vi "LifetimeImageglobal.vi"(1 "Palette Number (gray)":T2(ring), 4 "min tau value":dbl format="%.2f", 5 "max tau value":dbl format="%.2f", 6 "input Image array":u8[][](array[numeric]), 7 "error in":errorcluster, 8 "Enum":T1(ring)) -> (0 "title":string, 2 "error out":errorcluster, 3 "New Image":T3)   [LabVIEW 2009]
uses:
  <vilib>/vision/Image Controls.llb/IMAQ Image.ctl
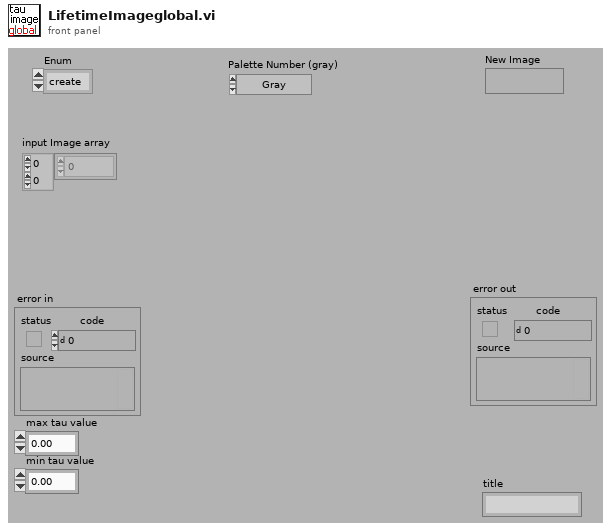
[diagram p1: front panel]
types:
  T1 = enum16{"create", "Input", "draw", "colorpal", "dump", "get", "kill"}
  T2 = enum32{"Gray", "Binary", "Gradient", "Rainbow", "Temperature"}
  T3 = typedef "IMAQ Image.ctl" = refnum<image>
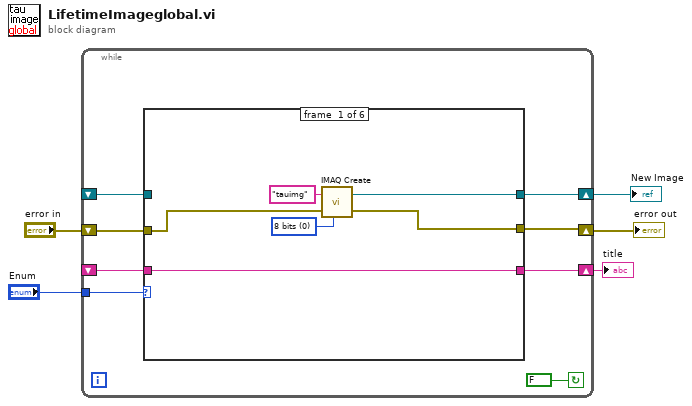
[diagram p0: block diagram]
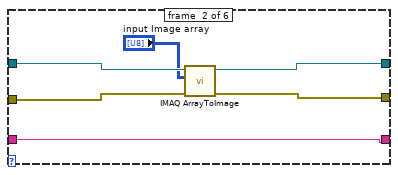
[diagram p2: hidden frame]
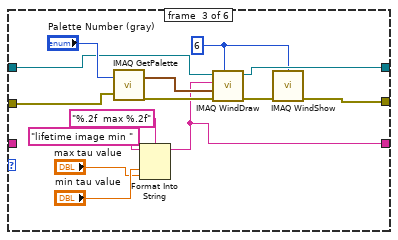
[diagram p3: hidden frame]
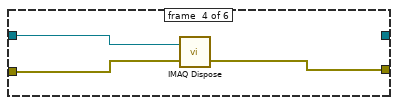
[diagram p4: hidden frame]
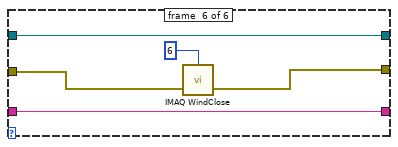
[diagram p6: hidden frame]
diagram:
  n1 = while {
    shift-right: [w11] -> w5
    shift-left: _ -> [w13]
    shift-right: [w10] -> w4
    shift-left: "error in" -> [w12]
    shift-right: [w9] -> w2
    shift-left: _ -> [w8]
    tunnel: "Enum" -> [w6]
    stop <- FALSE continue-if-true
    n2 = case shown="\"kill\"" w6 {
      tunnel: w13 -> [_ w23 w35 w42 w44 w49]
      tunnel: w12 -> [w16 w25 w39 w41 _ w47]
      tunnel: [w17 w22 w34 _ w44 w49] -> w11
      tunnel: [w15 w24 w32 w40 _ w46] -> w10
      tunnel: [w14 w20 w28 _ w43 w48] -> w9
      tunnel: w8 -> [w14 w20 _ _ w43 w48]
      frame #0 {
        w18 = u32 0 items=["8 bits", "16 bits", "Float", "Complex", "RGB", "HSL"] ("Image Type")
        n3 = call "IMAQ Create"("Image Name"="tauimg", "Image Type"=w18, "error in (no error)"=w16) -> ("New Image"=w17:T3, "error out"=w15:errorcluster)  [unwired: 2 in]
      }
      frame #1 {
        n4 = call "IMAQ ArrayToImage"("error in (no error)"=w25, "Image Pixels (U8)"="input Image array", "Image"=w23) -> ("error out"=w24:errorcluster, "Image Out"=w22:T3)  [unwired: 7 in]
      }
      frame #2 {
        w31 = 6 ("Window Number (0...15)")
        n5 = call "IMAQ GetPalette"("Palette Number (gray)"="Palette Number (gray)", "error in (no error)"=w39) -> ("Color Palette"=w36:cluster{"Red":u8, "Green":u8, "Blue":u8}[], "error out"=w37:errorcluster)  [unwired: 3 in]
        n6 = Format Into String(format string="%.2f  max %.2f", initial string="lifetime image min ", "min tau value", "max tau value") -> (resulting string=w28:string)  [unwired: 1 in, 1 out]
        n7 = call "IMAQ WindDraw"("Window Number (0...15)"=w31, "error in (no error)"=w37, "Color Palette"=w36, "Title"=w28, "Image"=w35) -> ("error out"=w33:errorcluster, "Image Out (duplicate)"=w34:T3)  [unwired: 5 in]
        n8 = call "IMAQ WindShow"("error in (no error)"=w33, "Window Number (0...15)"=w31) -> ("error out"=w32:errorcluster)  [unwired: 4 in, 2 out]
      }
      frame #3 {
        n9 = call "IMAQ Dispose"("Image"=w42, "error in (no error)"=w41) -> ("error out"=w40:errorcluster)  [unwired: 4 in]
      }
      frame #4 {
      }
      frame #5 {
        n10 = call "IMAQ WindClose"("Window Number (0...15)"=6, "error in (no error)"=w47) -> ("error out"=w46:errorcluster)  [unwired: 4 in]
      }
    }
  }
  "New Image" <- w5
  "error out" <- w4
  "title" <- w2
